vi "gyro -- async sweeper engine.vi"(11 "sweeper event pair":T4) -> ()   [LabVIEW 2020]
uses:
  gyro -- async sweeper parameters.ctl
  freq scan type.ctl
  show-win- control.ctl
  server talk-to-back pair.ctl
  server talkback message type.ctl
  server talkto message type.ctl
  publisher action.ctl
  data source action.ctl
  array - generate range.vi
  array -- sort 2D array -- Complex.vi/05c44075-957c-bc42-b6fa-2799d0bc0485.vi
  <vilib>/Array/Sort 2D Array - Pop Stack.vi
  <vilib>/Array/Sort 2D Array - Push Stack.vi
  array -- sort 2D array -- Complex.vi/05c44075-957c-bc42-b6fa-2799d0bc0485.vi/5dd0d2be-718e-c148-b8fa-e083cdba2843.vi
  array -- sort 2D array -- Complex.vi/05c44075-957c-bc42-b6fa-2799d0bc0485.vi/095795a0-771d-c341-9fed-d90d2e44c51c.vi
panel:
  in  "Tab Control":enum32{"Page 1", "Page 2"}(tab)
  out "got here":bool=TRUE
  in  "sweeper parameters":T1={"delay-circle(msec)"=0, "N"=300, "scan type"=enum."linear", "gamma factor"=1.5, "history length"=1}
  in  "win":T3={"cen (Hz)"=32757.83435625395, "win (Hz)"=134.34356253945762, "left (Hz)"=32690.66257498422, "right (Hz)"=32825.00613752368}
  out "progress":i32(slide) min=0 max=300 step=1 scale=0.0..300.0
  out "stopped?":bool=TRUE
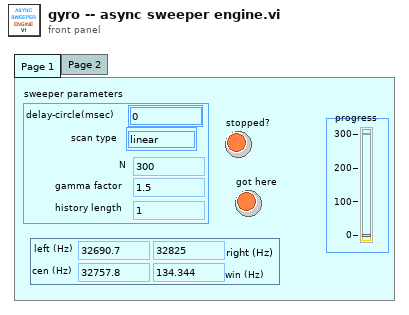
[diagram p1: front panel]
types:
  T1 = typedef "gyro -- async sweeper parameters.ctl" = cluster{"delay-circle(msec)":i64, "N":i64, "scan type":T2, "gamma factor":dbl, "history length":i64}
  T2 = typedef "freq scan type.ctl" = enum16{"linear", "arctan"}
  T3 = typedef "show-win- control.ctl" = cluster{"cen (Hz)":dbl, "win (Hz)":dbl, "left (Hz)":dbl, "right (Hz)":dbl}
  T4 = typedef "server talk-to-back pair.ctl" = cluster{"talkback event":refnum<user-event>, "talkto event":refnum<user-event>}
  T5 = typedef "publisher action.ctl" = enum16{"set", "get", "init", "check"}
  T6 = typedef "server talkback message type.ctl" = cluster{"message":enum16{"new", "void"}}
  T7 = typedef "data source action.ctl" = enum16{"set", "get", "init", "set-and-get", "init source"}
  T8 = enum16{"stop", "start", "update pars", "update request", "new", "launch", "exit", "get", "reset", "pause", "unpause"}
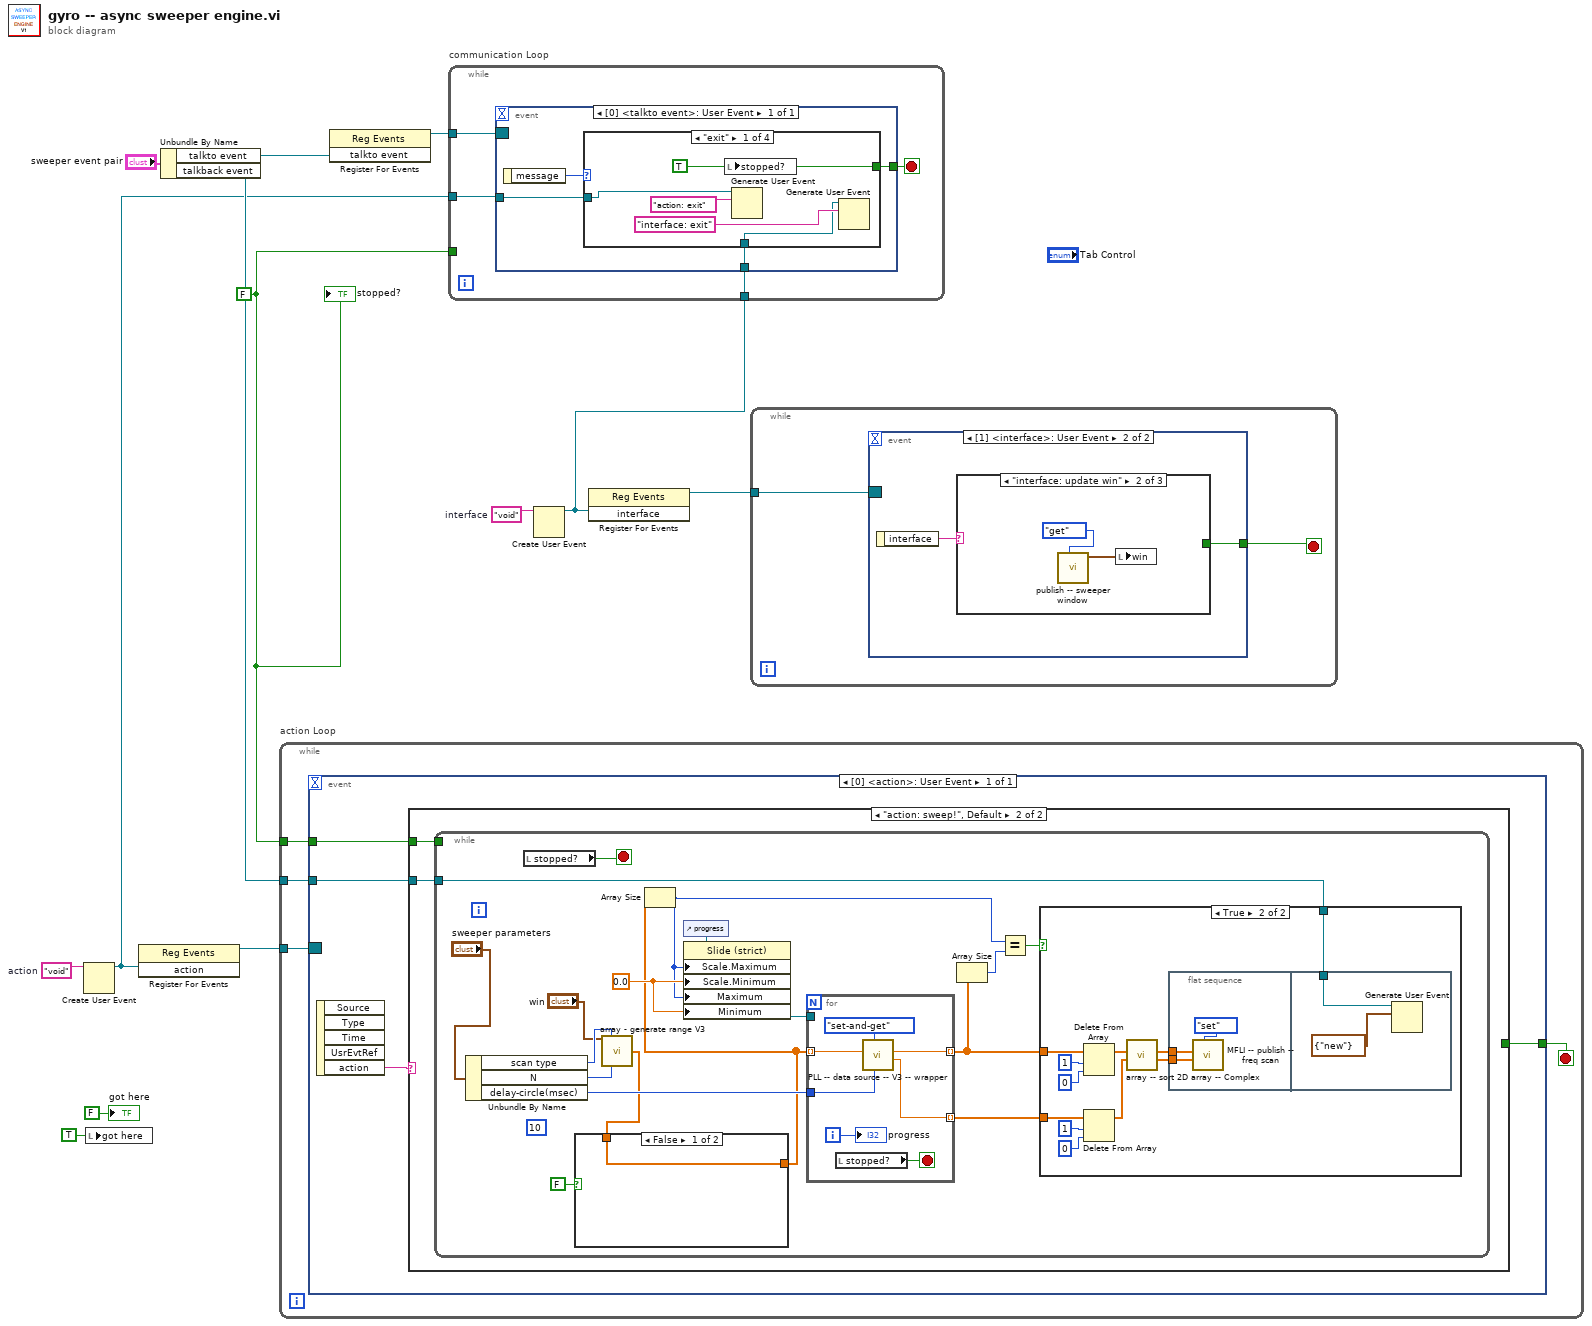
[diagram p0: block diagram]
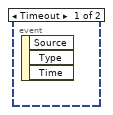
[diagram p2: hidden frame]
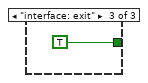
[diagram p4: hidden frame]
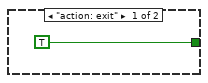
[diagram p5: hidden frame]
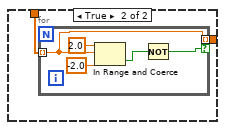
[diagram p6: hidden frame]
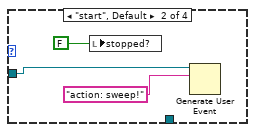
[diagram p8: hidden frame]
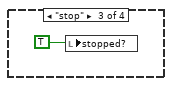
[diagram p9: hidden frame]
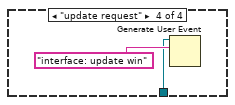
[diagram p10: hidden frame]
diagram:
  w3 = "void"  # interface
  w8 = "void"  # action
  w7 = FALSE ("stop!")
  n1 = Create User Event(user event datatype=w8) -> (user event=w6:refnum<user-event>)  [unwired: 1 in, 1 out]
  n2 = local write "got here"(TRUE ("got here")) -> ()
  n3 = register-events(w6) -> (reference out=w9:refnum<event-registration>)  [unwired: 2 in, 1 out]
  n4 = Unbundle By Name("sweeper event pair") -> ("talkto event"=w11:refnum<user-event>, "talkback event"=w10:refnum<user-event>)
  n5 = while "action Loop" {
    tunnel: w7 -> [w17]
    tunnel: w10 -> [w16]
    tunnel: w9 -> [w15]
    stop <- w14 stop-if-true
    n6 = event shown="[0] <action>: User Event" {
      selector: w15 -> [_]
      dyn-events: _ -> [_]
      timeout: _ -> [_]
      tunnel: w17 -> [w21]
      tunnel: w16 -> [w20]
      tunnel: [w18] -> w14
      event User Event {
        n7 = event-data() -> ("action"=w19:string)  [unwired: 1 in, 4 out]
        n8 = case shown="\"action: sweep!\", Default" w19 {
          tunnel: w21 -> [_ w24]
          tunnel: w20 -> [_ w23]
          tunnel: [TRUE ("stop!") _] -> w18
          frame "action: exit" {
          }
          frame "action: sweep!", Default {
            n9 = while {
              tunnel: w24 -> [_]
              tunnel: w23 -> [w40]
              stop <- w33 stop-if-true
              (unwired) 10 ("lower")
              w35 = 0.0 ("Scale.Range:Minimum")
              n10 = Unbundle By Name("sweeper parameters") -> ("scan type"=w39:T2, "N"=w28:i64, "delay-circle(msec)"=w38:i64)
              n11 = local read "stopped?"() -> (w33:bool)
              n12 = call "array - generate range V3.vi"("win"="win", "scan type"=w39, "N"=w28) -> ("Array"=w27:dbl[])  [unwired: 11 in, 1 out]
              n13 = case shown="False" FALSE {
                tunnel: w27 -> [w43 w45]
                tunnel: [w43 w44] -> w26
                frame False {
                }
                frame True {
                  n14 = for {
                    tunnel: w45 -> [w48] mode=indexing
                    tunnel: [w48] -> w44 mode=indexing if=w46
                    n15 = In Range and Coerce(upper limit=2.0, x=w48, lower limit=-2.0) -> (In Range?=w47:bool)  [unwired: 1 out]
                    n16 = Not(x=w47) -> (.not. x?=w46:bool)
                  }
                }
              }
              n17 = Array Size(array=w26) -> (size(s)=w29:i32)
              n18 = control-ref of="progress"() -> (w37:refnum<vi>)
              n19 = property class="Slide (strict)"(reference=w37, "Scale.Maximum"=w29, "Scale.Minimum"=w35, "Maximum"=w29, "Minimum"=w35) -> (reference out=w36:refnum<vi>)  [unwired: 1 in, 1 out]
              n20 = for {
                tunnel: w26 -> [w69] mode=indexing
                tunnel: w38 -> [w71]
                tunnel: [w73] -> w42 mode=indexing
                tunnel: [w72] -> w32 mode=indexing
                tunnel: w36 -> [_]
                i -> [w68]
                stop <- w67 stop-if-true
                n21 = local read "stopped?"() -> (w67:bool)
                n22 = call "PLL -- data source -- V3 -- wrapper.vi"("set-get delay (msec)"=w71, "data source action"=data_source_action."set-and-get", "Freq in (Hz)"=w69) -> ("z out (V)"=w73:cdb, "Freq out (Hz)"=w72:dbl)  [unwired: 6 in, 1 out]
                "progress" <- w68
              }
              n23 = Array Size(array=w32) -> (size(s)=w30:i32)
              n24 = Equal?(x=w29, y=w30) -> (x = y?=w31:bool)
              n25 = case shown="True" w31 {
                tunnel: w42 -> [_ w57]
                tunnel: w32 -> [_ w56]
                tunnel: w40 -> [_ w51]
                frame False {
                }
                frame True {
                  n26 = Delete From Array(array=w56, length=1, index=0) -> (array with subset deleted=w55:dbl[])  [unwired: 1 out]
                  n27 = Delete From Array(array=w57, length=1, index=0) -> (array with subset deleted=w54:cdb[])  [unwired: 1 out]
                  n28 = call "array -- sort 2D array -- Complex.vi"("z In"=w54, "freq IN"=w55) -> ("z out"=w52:cdb[], "freq out"=w53:dbl[])  [unwired: 8 in]
                  n29 = flat-sequence {
                    tunnel: w52 -> [w63]
                    tunnel: w53 -> [w62]
                    tunnel: w51 -> [w66]
                    frame #0 {
                      n30 = call "MFLI -- publish -- freq scan.vi"("publisher action"=publisher_action."set", "Voltage IN (V)"=w63, "Freq IN (Hz)"=w62) -> ()  [unwired: 7 in, 2 out]
                    }
                    frame #1 {
                      n31 = Generate User Event(user event=w66, event data cluster=T6 {"message"=enum."new"} ("event data")) -> ()  [unwired: 2 in, 2 out]
                    }
                  }
                }
              }
            }
          }
        }
      }
    }
  }
  n32 = register-events(w11) -> (reference out=w13:refnum<event-registration>)  [unwired: 2 in, 1 out]
  n33 = Create User Event(user event datatype=w3) -> (user event=w1:refnum<user-event>)  [unwired: 1 in, 1 out]
  n34 = while "communication Loop" {
    tunnel: w13 -> [w77]
    tunnel: w7 -> [_]
    tunnel: w6 -> [w75]
    tunnel: w1 -> [w74]
    stop <- w76 stop-if-true
    n35 = event shown="[0] <talkto event>: User Event" {
      selector: w77 -> [_]
      dyn-events: _ -> [_]
      timeout: _ -> [_]
      tunnel: [w81] -> w76
      tunnel: w75 -> [w79]
      tunnel: w74 -> [w78]
      event User Event {
        n36 = event-data() -> ("message"=w80:T8)  [unwired: 1 in]
        n37 = case shown="\"exit\"" w80 {
          tunnel: [w86 _ _ _] -> w81
          tunnel: w79 -> [w85 w88 _ _]
          tunnel: w78 -> [w82 _ _ w91]
          frame "exit" {
            w86 = TRUE ("stop!")
            n38 = local write "stopped?"(w86) -> ()
            n39 = Generate User Event(user event=w85, event data cluster="action: exit" ("event data")) -> ()  [unwired: 2 in, 2 out]
            n40 = Generate User Event(user event=w82, event data cluster="interface: exit" ("event data")) -> ()  [unwired: 2 in, 2 out]
          }
          frame "start", Default {
            n41 = local write "stopped?"(FALSE ("stop!")) -> ()
            n42 = Generate User Event(user event=w88, event data cluster="action: sweep!" ("event data")) -> ()  [unwired: 2 in, 2 out]
          }
          frame "stop" {
            n43 = local write "stopped?"(TRUE ("stop!")) -> ()
          }
          frame "update request" {
            n44 = Generate User Event(user event=w91, event data cluster="interface: update win" ("event data")) -> ()  [unwired: 2 in, 2 out]
          }
        }
      }
    }
  }
  n45 = register-events(w1) -> (reference out=w2:refnum<event-registration>)  [unwired: 2 in, 1 out]
  n46 = while {
    tunnel: w2 -> [w94]
    stop <- w93 stop-if-true
    n47 = event shown="[1] <interface>: User Event" {
      selector: w94 -> [_ _]
      dyn-events: _ -> [_ _]
      timeout: _ -> [_ _]
      tunnel: [_ w95] -> w93
      event Timeout {
        n48 = event-data() -> ()  [unwired: 1 in, 3 out]
      }
      event User Event {
        n49 = event-data() -> ("interface"=w96:string)  [unwired: 1 in]
        n50 = case shown="\"interface: update win\"" w96 {
          tunnel: [_ _ TRUE] -> w95
          frame "False", Default {
          }
          frame "interface: update win" {
            n51 = call "publish -- sweeper window.vi"("publisher action"=publisher_action."get") -> ("win OUT"=w98:T3)  [unwired: 10 in]
            n52 = local write "win"(w98) -> ()
          }
          frame "interface: exit" {
          }
        }
      }
    }
  }
  "stopped?" <- w7
  "got here" <- FALSE ("got here")
